vi "3-2.vi"() -> ()   [LabVIEW 2022 SP3, in "AoC22.lvlib"]
uses:
  AoC22.lvlib
  3c698400-f7ac-4985-91dc-36f0f990e279.vi
  6b0cb146-09b0-49f1-b303-3844e7943c27.vi
  <vilib>/IlluminatedG/lv-stream/Stream.lvlib
panel:
  out "sum":i32
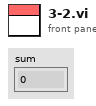
[diagram p1: front panel]
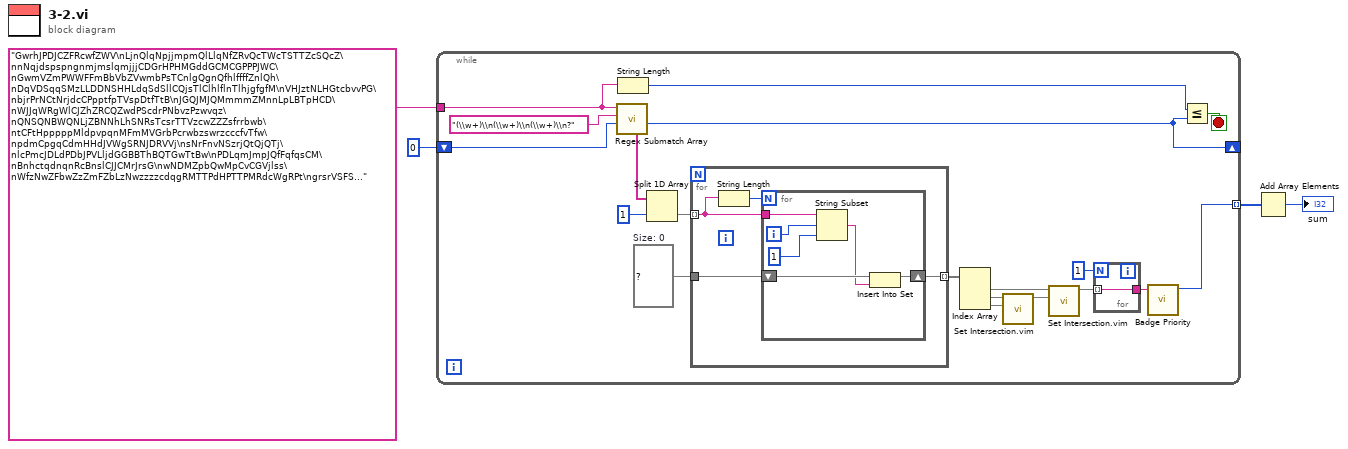
[diagram p0: block diagram]
diagram:
  n1 = while {
    tunnel: "GwrhJPDJCZFRcwfZWV\nLjnQlqNpjjmpmQlLlqNfZRvQcTWcTSTTZcSQcZ\nnNqjdspspngnmjmslqmjjjCDGrHPHMGddGCMCGPPPJWC\nGwmVZmPWWFFmBbVbZVwmbPsTCnlgQgnQfhlffffZnlQh\nDqVDSqqSMzLLDDNSHHLdqSdSllCQjsTlClhlflnTlhjgfgfM\nVHJztNLHGtcbvvPG\nbjrPrNCtNrjdcCPpptfpTVspDtfTtB\nJGQJMJQMmmmZMnnLpLBTpHCD\nWJJqWRgWlCJZhZRCQZwdPScdrPNbvzPzwvqz\nQNSQNBWQNLjZBNNhLhSNRsTcsrTTVzcwZZZsfrrbwb\ntCFtHpppppMldpvpqnMFmMVGrbPcrwbzswrzcccfvTfw\npdmCpgqCdmHHdJVWgSRNJDRVVj\nsNrFnvNSzrjQtQjQTj\nlcPmcJDLdPDbJPVLljdGGBBThBQTGwTtBw\nPDLqmJmpJQfFqfqsCM\nBnhctqdnqnRcBnslCJJCMrJrsG\nwNDMZpbQwMpCvCGVjlss\nWfzNwZFbwZzZmFZbLzNwzzzzcdqgRMTTPdHPTTPMRdcWgRPt\ngrsrVSFS..." -> [w18]
    shift-right: [w16] -> _
    shift-left: 0 -> [w22]
    tunnel: [w5] -> w2 mode=indexing
    stop <- w15 stop-if-true
    w14 = set{string} {}  # Size: 0
    n2 = call <vilib>:"Regex Submatch Array.vi"("offset (0)"=w22, "regular expression"="(\\w+)\\n(\\w+)\\n(\\w+)\\n?", "string"=w18) -> ("offset past match"=w16:i32, "matches"=w21:string[])  [unwired: 6 in, 1 out]
    n3 = String Length(string=w18) -> (length=w17:i32)
    n4 = Split 1D Array(array=w21, index=1) -> (second subarray=w19:string[])  [unwired: 1 out]
    n5 = for {
      tunnel: w19 -> [w28] mode=indexing
      tunnel: w14 -> [w26]
      tunnel: [w25] -> w13 mode=indexing
      n6 = String Length(string=w28) -> (length=w27:i32)
      n7 = for {
        N: w27 -> [_]
        tunnel: w28 -> [w34]
        shift-right: [w29] -> w25
        shift-left: w26 -> [w31]
        i -> [w33]
        n8 = String Subset(string=w34, offset (0)=w33, length (rest)=1 ("length (rest)")) -> (substring=w30:string)
        n9 = Insert Into Set(10:w30, 11:w31) -> (3:w29:set{string})  [unwired: 1 out]
      }
    }
    n10 = Index Array(array=w13) -> (element #1=w10:set{string}, element #2=w12:set{string}, element #3=w11:set{string})  [unwired: 3 in]
    n11 = call "Set Intersection.vim"("set 2"=w11, "set 1"=w12) -> ("intersection"=w9:set{string})  [unwired: 9 in]
    n12 = call "Set Intersection.vim"("set 2"=w9, "set 1"=w10) -> ("intersection"=w7:set{string})  [unwired: 9 in]
    n13 = for {
      N: 1 -> [_]
      tunnel: w7 -> [w24] mode=indexing
      tunnel: [w24] -> w6
    }
    n14 = call "Badge Priority.vi"("Code"=w6) -> ("Priority"=w5:i32)  [unwired: 10 in]
    n15 = Less Or Equal?(x=w17, y=w16) -> (x <= y?=w15:bool)
  }
  n16 = Add Array Elements(numeric array=w2) -> (sum=→"sum":i32)
